vi "ep_Hilbert Demodulation.vi"(6 "previous state":T1, 7 "reset? (F)":bool, 8 "error in (no error)":errorcluster, 9 "filter information":cluster{"coefficients":dbl[], "delay":i32}, 11 "signal":dbl[](array[numeric])) -> (0 "error out":errorcluster, 3 "demodulated signal":dbl[](array[numeric]), 4 "next state":T1)   [LabVIEW 2014, in "NI_EP_Motor Monitoring.lvlib"]
uses:
  <vilib>/addons/Electrical Power/Motor Monitoring/NI_EP_Motor Monitoring.lvlib
  <vilib>/Analysis/3filter.llb/FIR Filter with I.C. (DBL).vi
  <vilib>/Analysis/NI_AALBase.lvlib
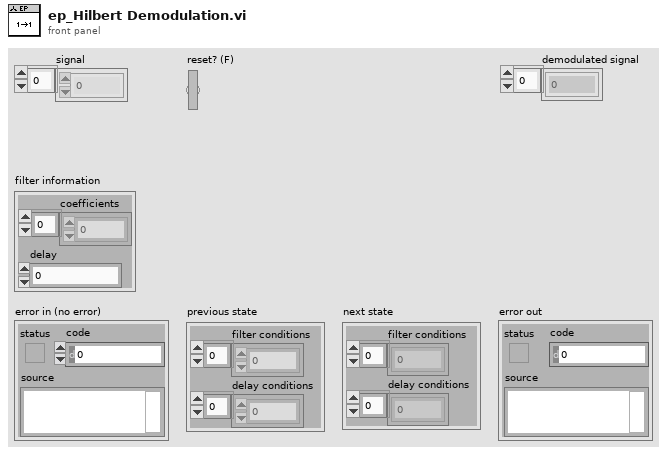
[diagram p1: front panel]
types:
  T1 = cluster{"filter conditions":dbl[], "delay conditions":dbl[]}
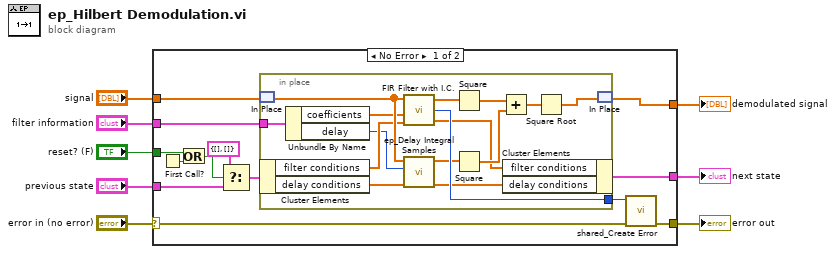
[diagram p0: block diagram]
diagram:
  n1 = case shown="No Error" "error in (no error)" {
    selector: "error in (no error)" -> [w20 w37]
    tunnel: "signal" -> [w11 _]
    tunnel: [w18 w37] -> w7
    tunnel: "filter information" -> [w19 _]
    tunnel: "previous state" -> [w13 _]
    tunnel: [w9 _] -> w3
    tunnel: [w10 _] -> w2
    tunnel: "reset? (F)" -> [w16 _]
    frame No Error {
      n2 = First Call?() -> (First Call?: T/F=w17:bool)
      n3 = Or(x=w16, y=w17) -> (x .or. y?=w15:bool)
      n4 = Select(t=T1 {"filter conditions"=[], "delay conditions"=[]} ("previous conditions"), s=w15, f=w13) -> (s? t:f=w12:T1)
      n5 = in-place {
        in-place-border: [w36] -> w21
        in-place-border: w19 -> [w24]
        n6 = in-place-match #1(w11) -> (w27:dbl[])
        n7 = in-place-cluster #2(w12) -> ("filter conditions"=w25:dbl[], "delay conditions"=w30:dbl[])
        n8 = Unbundle By Name(w24) -> ("coefficients"=w23:dbl[], "delay"=w22:i32)
        n9 = call-poly <vilib>:"FIR Filter with I.C..vi"("Initial X Conditions"=w25, "FIR Coefficients"=w23, "X"=w27) -> ("Final X Conditions"=w28:dbl[], "error"=w36:i32, "Filtered X"=w35:dbl[])  [unwired: 5 in]
        n10 = call <vilib>:"ep_Delay Integral Samples.vi"("state in"=w30, "delay"=w22, "signal in"=w27) -> ("state out"=w29:dbl[], "signal out"=w34:dbl[])  [unwired: 7 in]
        n11 = Square(x=w35) -> (x^2=w33:dbl[])
        n12 = Square(x=w34) -> (x^2=w32:dbl[])
        n13 = Add(x=w33, y=w32) -> (x+y=w31:dbl[])
        n14 = in-place-cluster #2("filter conditions"=w28, "delay conditions"=w29) -> (w9:T1)
        n15 = Square Root(x=w31) -> (sqrt(x)=w26:dbl[])
        n16 = in-place-match #1(w26) -> (w10:dbl[])
      }
      n17 = call <vilib>:"shared_Create Error.vi"("error in (no error)"=w20, "error code (0)"=w21) -> ("error out"=w18:errorcluster)  [unwired: 9 in]
    }
    frame Error {
    }
  }
  "demodulated signal" <- w2
  "error out" <- w7
  "next state" <- w3
